vi "AOL Z Cal-Message switch.vi"(8 "error in (no error)":errorcluster, 11 "State":T1=enum."Select cal mode") -> (0 "error out":errorcluster)   [LabVIEW 2020]
uses:
  Typedefs/AOL Z cal wizard states.ctl
  Globals/gl_Calibration globals.vi
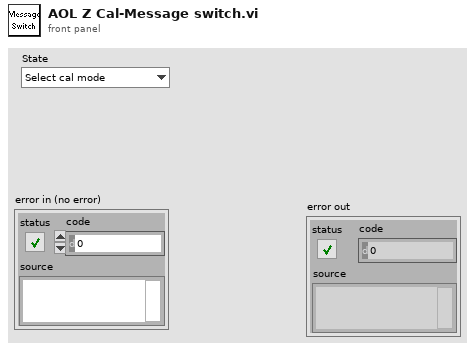
[diagram p1: front panel]
types:
  T1 = typedef "AOL Z cal wizard states.ctl" = enum16{"Idle", "Select cal mode", "Select cal points", "Select channel", "Start calibration"}
  T2 = typedef "Pre-AOL Z wizard refs.ctl" = cluster{"VI's reference":refnum<vi>, "Calibration Mode":refnum<vi>, "Cal points":refnum<vi>, "Channel Selector":refnum<vi>, "Message":refnum<vi>, "Back":refnum<vi>, "Next":refnum<vi>, "Power meter AI":refnum<vi>, "2D Picture":refnum<vi>, "Note":refnum<vi>}
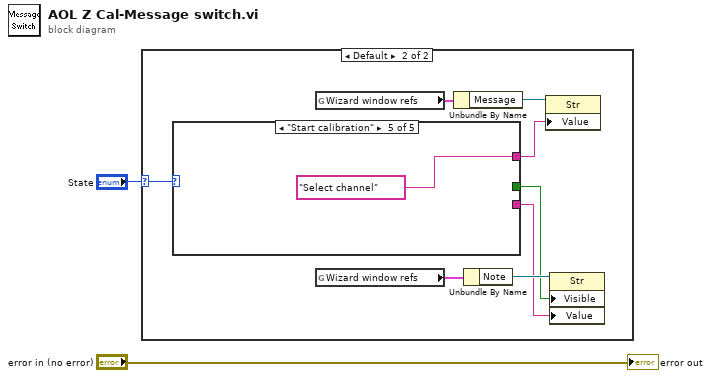
[diagram p0: block diagram]
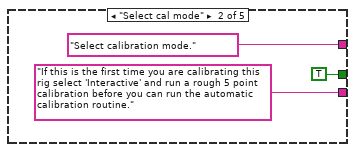
[diagram p4: hidden frame]
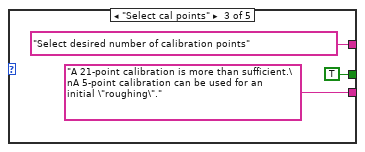
[diagram p5: hidden frame]
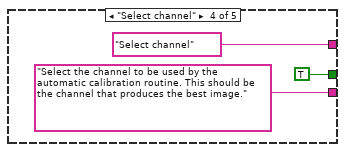
[diagram p6: hidden frame]
diagram:
  n1 = case shown="Default" "State" {
    selector: "State" -> [_ w7]
    frame "Idle" {
    }
    frame Default {
      n2 = case shown="\"Start calibration\"" w7 {
        tunnel: [_ "Select calibration mode." ("Value") "Select desired number of calibration points" ("Value") "Select channel" ("Value") "Select channel" ("Value")] -> w8
        tunnel: [_ "If this is the first time you are calibrating this rig select 'Interactive' and run a rough 5 point calibration before you can run the automatic calibration routine." ("Value") "A 21-point calibration is more than sufficient.\nA 5-point calibration can be used for an initial \"roughing\"." ("Value") "Select the channel to be used by the automatic calibration routine. This should be the channel that produces the best image." ("Value") _] -> w4
        tunnel: [_ TRUE TRUE TRUE _] -> w3
        frame Default {
        }
        frame "Select cal mode" {
        }
        frame "Select cal points" {
        }
        frame "Select channel" {
        }
        frame "Start calibration" {
        }
      }
      n3 = global read "gl_Calibration globals.vi" "Wizard window refs"() -> (w9:T2)
      n4 = global read "gl_Calibration globals.vi" "Wizard window refs"() -> (w6:T2)
      n5 = Unbundle By Name(w9) -> ("Message"=w10:refnum<vi>)
      n6 = Unbundle By Name(w6) -> ("Note"=w5:refnum<vi>)
      n7 = property on="Property Node" class="Str"(reference=w10, "Value"=w8) -> ()  [unwired: 1 in, 2 out]
      n8 = property on="Property Node" class="Str"(reference=w5, "Visible"=w3, "Value"=w4) -> ()  [unwired: 1 in, 2 out]
    }
  }
  "error out" <- "error in (no error)"
